vi "Log State.vi"(8 "error in (no error)":errorcluster, 10 "state":T1=enum."Start", 11 "Plugin Thread in":refnum<class "Plugin Thread.lvclass">) -> (0 "error out":errorcluster, 3 "Plugin Thread out":refnum<class "Plugin Thread.lvclass">)   [LabVIEW 2019, in "DSF Core.lvlib" / "Plugin Thread.lvclass"]
uses:
  Plugin Thread.lvclass
  C:/Dev/GitHub/niveristand-data-sharing-framework-custom-device/Core/Classes/Thread/Thread.lvclass
  Interface/Plugin/Command.ctl
  Thread.lvclass/Thread.ctl
  Pointers/Error/Error Pointer.lvclass/Error Pointer.ctl
  <vilib>/NI/Memory Manager/Classes/Pointer/Pointer.lvclass/Pointer.ctl
  Plugin Thread.lvclass/Plugin Thread.ctl
  Interface/Logging/Parameters.ctl
  Interface/Logging/Plugin State Parameters.ctl
  Interface/Logging/Command.ctl
  Interface/Logging/Command Data.ctl
  Interface/Interface.lvclass/Interface.ctl
  Interface/Logging/Send Logging Command.vi
  Interface/Send Command.vi
  Interface/Errors.vi
  Interface/Dispatcher/Command Timeout.vi
  Interface/Write RT FIFO.vi
  Interface/New Interface Error.vi
  <vilib>/NI/Memory Manager/Classes/Pointer/Write.vi
  <vilib>/NI/Memory Manager/Classes/Pointer/Write 1D U8.vi
  <vilib>/NI/Memory Manager/Classes/Pointer/Clear.vi
  Pointers/Error/Get Power Of 2.vi
  <vilib>/NI/Memory Manager/VIs/New Error Cluster.vi
  <vilib>/NI/Memory Manager/VIs/New Error Cluster (512B).vi
  <vilib>/NI/Memory Manager/VIs/Set Error Code.vi
  <vilib>/NI/Memory Manager/VIs/Set Error Status.vi
  <vilib>/NI/Memory Manager/VIs/Set Error Source.vi
  <vilib>/NI/Memory Manager/VIs/Write String to Source.vi
  Interface/Interface Error Info.vi
  <vilib>/NI/Memory Manager/Classes/Pointer/Write (No Check).vi
  <vilib>/NI/Memory Manager/Classes/Pointer/Write (No Check) 1D U8.vi
  <vilib>/NI/Memory Manager/Classes/Pointer/Check Move.vi
  <vilib>/NI/Memory Manager/Classes/Pointer/Check Null Pointer.vi
  <vilib>/NI/Memory Manager/Classes/Pointer/Clear (No Check).vi
  <vilib>/NI/Memory Manager/Classes/Pointer/Check Length.vi
  VIs/Constants/Constants.vi
  VIs/Constants/Base Error Code.vi
  Interface/Interface Error Offset.vi
  <vilib>/NI/Memory Manager/Classes/Pointer/Check Count.vi
  <vilib>/NI/Memory Manager/Classes/Pointer/Check Bounds (Power of 2).vi
  <vilib>/NI/Memory Manager/Classes/Pointer/Errors.vi
  <vilib>/NI/Memory Manager/Classes/Pointer/Null Pointer.vi
  <vilib>/NI/Memory Manager/Classes/Pointer/Is Null.vi
  <vilib>/NI/Memory Manager/Classes/Pointer/Get Size.vi
  <vilib>/NI/Memory Manager/Classes/Pointer/Check Bounds (Pointer).vi
  <vilib>/NI/Memory Manager/Classes/Pointer/Out of Bounds.vi
  <vilib>/NI/Memory Manager/Classes/Pointer/Check Bounds.vi
  <vilib>/NI/Memory Manager/Classes/Pointer/Create Error.vi
  <vilib>/NI/Memory Manager/Classes/Pointer/Write Pointer Size to Error.vi
  <vilib>/NI/Memory Manager/VIs/Write Numeric to Source.vi
  <vilib>/NI/Memory Manager/VIs/Write Numeric Scalar to Source (Base10 U64).vi
  <vilib>/NI/Memory Manager/Classes/Pointer/Check Bounds (Buffer).vi
  <vilib>/NI/Memory Manager/Constants/Constants.vi
  <vilib>/NI/Memory Manager/Constants/Library Name.vi
  <vilib>/NI/Memory Manager/Classes/Pointer/Pointer Error Info.vi
  <vilib>/NI/Memory Manager/Constants/Pointer Class Name.vi
  <vilib>/NI/Memory Manager/Classes/Pointer/Buffer Underflow.vi
  Pointers/Error/Error Pointer.lvclass
  C:/Program Files (x86)/National Instruments/LabVIEW 2019/vi.lib/NI/Memory Manager/Classes/Pointer/Pointer.lvclass
  Interface/Logging/Logging Interface.lvclass
  C:/Dev/GitHub/niveristand-data-sharing-framework-custom-device/Core/Classes/Interface/Interface.lvclass
  VIs/VI Name.vi
  Interface/Plugin/Plugin Interface.lvclass
  Thread.lvclass
  <vilib>/NI/Memory Manager/Classes/Pointer/Pointer.lvclass
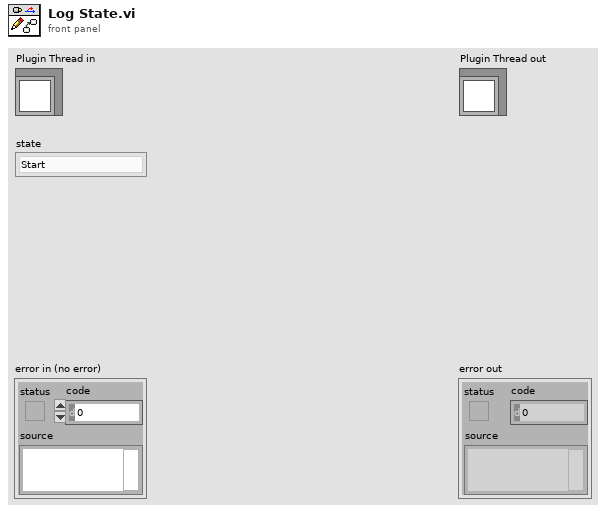
[diagram p1: front panel]
types:
  T1 = typedef "DSF Core.lvlib/Plugin Interface.lvclass/Command.ctl" = enum8{"Idle", "Start", "Set Inline Buffer", "Rx", "Tx", "Shutdown", "Error"}
  T2 = typedef "DSF Core.lvlib/Logging Interface.lvclass/Parameters.ctl" = cluster{"arg1":u64, "arg2":u64}
  T3 = typedef "DSF Core.lvlib/Logging Interface.lvclass/Plugin State Parameters.ctl" = cluster{"state":T1, "Plugin ID":u8, "Thread ID":u8, "unused 0":u8, "unused 1":i32, "error pointer":u64}
  T4 = typedef "DSF Core.lvlib/Logging Interface.lvclass/Command.ctl" = enum8{"Idle", "Start", "Log Framework State", "Log Plugin State", "Log Dispatcher State", "Shutdown"}
  T5 = typedef "DSF Core.lvlib/Logging Interface.lvclass/Command Data.ctl" = cluster{"Command":T4, "Parameters":T2}
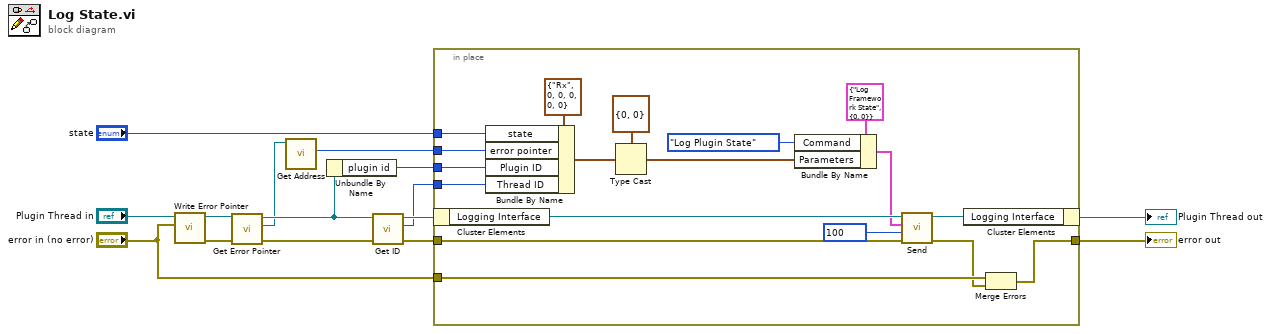
[diagram p0: block diagram]
diagram:
  n1 = call "Write Error Pointer.vi"("error"="error in (no error)", "Thread in"="Plugin Thread in") -> ("error out"=w12:errorcluster, "Thread out"=w11:refnum<class "Plugin Thread.lvclass">)  [unwired: 8 in]
  n2 = call "Get Error Pointer.vi"("Thread in"=w11) -> ("error pointer"=w2:refnum<class "Error Pointer.lvclass">, "Thread out"=w9:refnum<class "Plugin Thread.lvclass">)  [unwired: 9 in]
  n3 = call <vilib>:"Get Address.vi"("Pointer in"=w2) -> ("address"=w13:u64)  [unwired: 9 in, 1 out]
  n4 = Unbundle By Name(w9) -> ("plugin id"=w10:i32)
  n5 = call "Get ID.vi"("Thread in"=w9) -> ("ID"=w7:i32, "Thread out"=w8:refnum<class "Plugin Thread.lvclass">)  [unwired: 9 in]
  n6 = in-place {
    in-place-border: [w14] -> w4
    in-place-border: w12 -> [w26]
    in-place-border: "state" -> [w21]
    in-place-border: w13 -> [w19]
    in-place-border: w10 -> [w18]
    in-place-border: w7 -> [w17]
    in-place-border: "error in (no error)" -> [w16]
    n7 = in-place-cluster #1(w8) -> ("Logging Interface"=w31:refnum<class "Logging Interface.lvclass">)
    n8 = Bundle By Name(cluster=T3 {"state"=enum."Rx", "Plugin ID"=0, "Thread ID"=0, "unused 0"=0, "unused 1"=0, "error pointer"=0} ("Parameters"), "state"=w21, "error pointer"=w19, "Plugin ID"=w18, "Thread ID"=w17) -> (w24:T3)
    n9 = Type Cast(type=T2 {"arg1"=0, "arg2"=0} ("Parameters"), x=w24) -> (*(type *) &x=w22:T2)
    n10 = Bundle By Name(cluster=T5 {"Command"=enum."Log Framework State", "Parameters"={"arg1"=0, "arg2"=0}} ("command"), "Command"=Command."Log Plugin State", "Parameters"=w22) -> (w28:T5)
    n11 = call-poly "Send.vi"("error in (no error)"=w26, "timeout in ms (0)"=100, "command"=w28, "Logging Interface in"=w31) -> ("error out"=w15:errorcluster, "Logging Interface out"=w27:refnum<class "Logging Interface.lvclass">)  [unwired: 6 in]
    n12 = in-place-cluster #1("Logging Interface"=w27) -> (→"Plugin Thread out":refnum<class "Plugin Thread.lvclass">)
    n13 = Merge Errors(w16, w15) -> (w14:errorcluster)
  }
  "error out" <- w4
